vi "test4.vi"() -> ()   [LabVIEW 2020]
uses:
  <vilib>/Platform/TimedLoop/XDataNode/timing_clust.ctl
  <vilib>/Platform/TimedLoop/XDataNode/nitl_modes.ctl
  <vilib>/Platform/TimedLoop/XDataNode/wakeup.ctl
  37583fcc-cec8-480d-a6d0-1da09da3d0dd.vi
  <vilib>/platform/TimedLoop/XDataNode/XDataNode.xnode
  <vilib>/Platform/TimedLoop/XDataNode/XDNodeRunTimeDep.lvlib
panel:
  out "Tank":dbl(slide) scale=0.0..1.0
  out "Current XY":cluster{"X":dbl, "Y":dbl}
  out "XY Graph":cluster{dbl[], dbl[]}[](graph)
  out "Move Time":u32
  out "Distance":dbl
  out "Start Time":u32
  out "Start XY":cluster{"X":dbl, "Y":dbl}
  out "Target XY":cluster{"X":dbl, "Y":dbl}
  out "Stopped":bool
  in  "Stop":bool
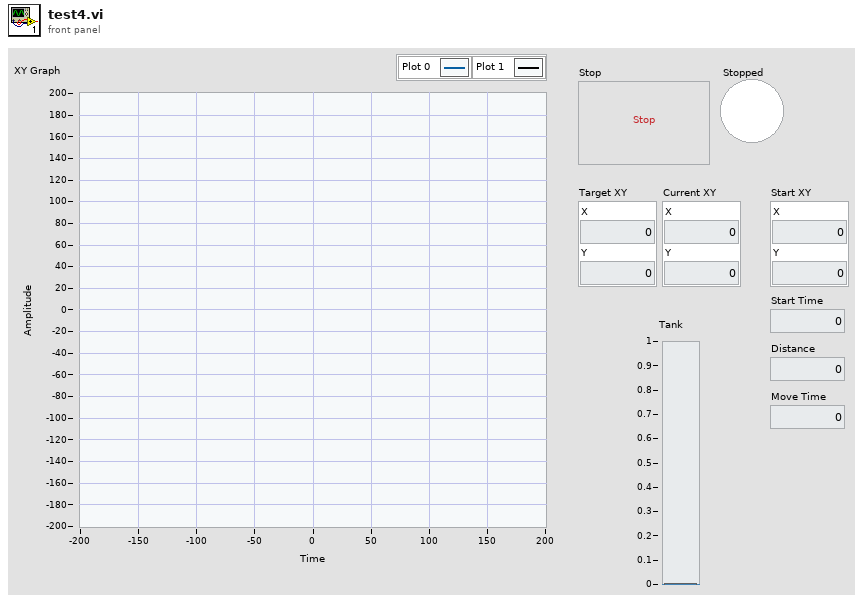
[diagram p1: front panel]
types:
  T1 = typedef "XDNodeRunTimeDep.lvlib/timing_clust.ctl" = cluster{"Expected End [f-1]":u64, "Actual End [f-1]":u64, "Finished Late? [f-1]":bool, "Expected End [i-1]":u64, "Actual End [i-1]":u64, "Finished Late? [i-1]":bool, "Expected Start [i]":u64, "Actual Start [i]":u64, "Expected Start [f]":u64, "Actual Start [f]":u64, "Source Name":string, "Structure Name":string, "Period":i64, "Deadline":i64, "Offset":i64, "Start":i64, "Priority":i32, "Timeout":i32, "Mode":T2, "Wakeup Reason":T3, "Error":errorcluster, "Source Type":string, "Secondary Source Type":string, "Global End Time":u64, "Global Start Time":u64, "Frame Duration":u64, "Iteration Duration":u64, "Assigned CPU":i32, "I/O Scan Engine Mode":u32}
  T2 = typedef "XDNodeRunTimeDep.lvlib/nitl_modes.ctl" = enum32{"No Change", "Process missed periods, maintain original phase", "Discard missed periods, maintain original phase", "Process missed periods, ignore original phase", "Discard missed periods, ignore original phase"}
  T3 = typedef "XDNodeRunTimeDep.lvlib/wakeup.ctl" = enum32{"Normal", "Aborted", "Asynchronous wakeup", "Timing source error", "Timed loop error", "Timeout"}
  T4 = typedef "LVPoint32TypeDef.ctl" = cluster{"Horizontal":i32, "Vertical":i32}
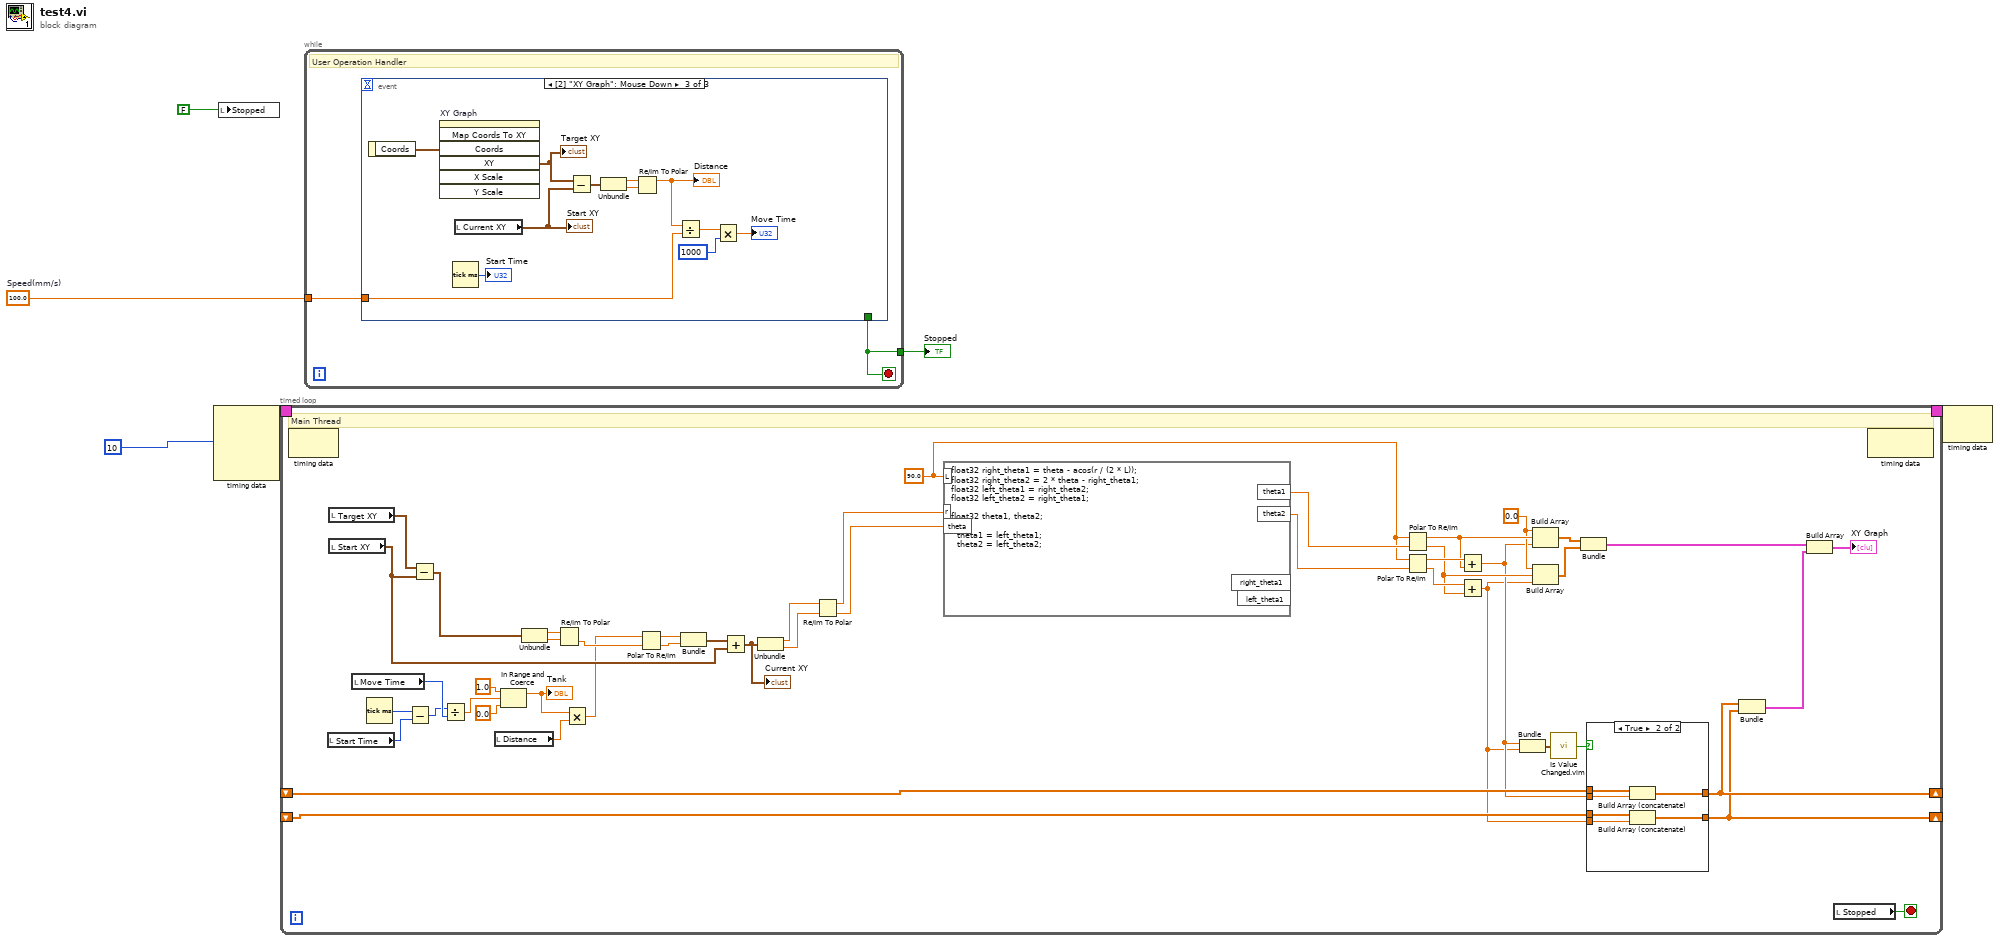
[diagram p0: block diagram]
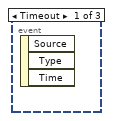
[diagram p3: hidden frame]
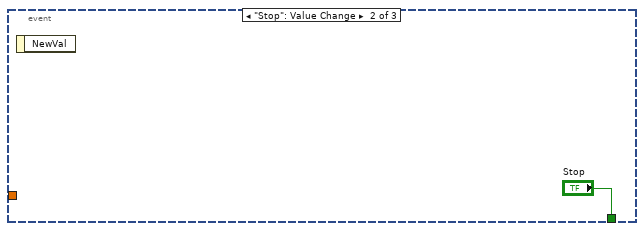
[diagram p4: hidden frame]
diagram:
  w1 = 100.0  # Speed(mm/s)
  n1 = node-c288(i64 10 ("Period")) -> (w6:T1)  [unwired: 3 in]
  n2 = local write "Stopped"(FALSE ("Stopped")) -> ()
  n3 = timed-loop {
    timing: w6 -> [_]
    timing-out: [_] -> w5
    shift-right: [w15] -> _
    shift-left: _ -> [w22]
    shift-right: [w14] -> _
    shift-left: _ -> [w21]
    stop <- w52 stop-if-true
    w27 = 0.0 ("element")
    w24 = 90.0 ("input variable")
    # "Main Thread"
    n4 = node-c288() -> ()  [unwired: 1 in, 1 out]
    n5 = local read "Start Time"() -> (w50:u32)
    n6 = local read "Target XY"() -> (w49:cluster{"X":dbl, "Y":dbl})
    n7 = local read "Start XY"() -> (w40:cluster{"X":dbl, "Y":dbl})
    n8 = local read "Move Time"() -> (w36:u32)
    n9 = Tick Count (ms)() -> (millisecond timer value=w51:u32)
    n10 = Subtract(x=w51, y=w50) -> (x-y=w11:u32)
    n11 = Subtract(x=w49, y=w40) -> (x-y=w47:cluster{"X":dbl, "Y":dbl})
    n12 = Divide(x=w11, y=w36) -> (x/y=w10:dbl)
    n13 = local read "Distance"() -> (w48:dbl)
    n14 = In Range and Coerce(upper limit=1.0 ("lower limit"), x=w10, lower limit=0.0) -> (coerced(x)=w7:dbl)  [unwired: 1 out]
    "Tank" <- w7
    n15 = Unbundle(w47) -> ("X"=w46:dbl, "Y"=w45:dbl)
    n16 = Re/Im To Polar(2:w45, 3:w46) -> (0:w44:dbl)  [unwired: 1 out]
    n17 = Multiply(x=w7, y=w48) -> (x*y=w35:dbl)
    n18 = Polar To Re/Im(2:w44, 3:w35) -> (0:w42:dbl, 1:w43:dbl)
    n19 = Bundle(w43, w42) -> (w41:cluster{dbl, dbl})  [unwired: 1 in]
    n20 = Add(x=w41, y=w40) -> (x+y=w23:cluster{dbl, dbl})
    "Current XY" <- w23
    n21 = Unbundle(w23) -> (w39:dbl, w38:dbl)
    n22 = Re/Im To Polar(2:w38, 3:w39) -> (0:w37:dbl, 1:w34:dbl)
    n23 = formula code="float32 right_theta1 = theta - acos(r / (2 * L));\nfloat32 right_theta2 = 2 * theta - right_theta1;\nfloat32 left_theta1 = right_theta2;\nfloat32 left_theta2 = right_theta1;\n\nfloat32 theta1, theta2;\n\n  theta1 = left_theta1;\n  theta2 = left_theta2;"("r"=w34, "theta"=w37, "L"=w24) -> ("theta1"=w26:sgl, "theta2"=w25:sgl)  [unwired: 2 out]
    n24 = Polar To Re/Im(2:w26, 3:w24) -> (0:w30:dbl, 1:w31:dbl)
    n25 = Polar To Re/Im(2:w25, 3:w24) -> (0:w32:dbl, 1:w33:dbl)
    n26 = Add(x=w33, y=w31) -> (x+y=w20:dbl)
    n27 = Add(x=w32, y=w30) -> (x+y=w19:dbl)
    n28 = Bundle(w20, w19) -> (w18:cluster{dbl, dbl})  [unwired: 1 in]
    n29 = Build Array(w27, w31, w20) -> (w29:dbl[])
    n30 = Build Array(w27, w30, w19) -> (w28:dbl[])
    n31 = call "Is Value Changed.vim"("value"=w18) -> ("changed or first call?"=w17:bool)
    n32 = Bundle(w29, w28) -> (w16:cluster{dbl[], dbl[]})  [unwired: 1 in]
    n33 = case shown="True" w17 {
      tunnel: w20 -> [_ w60]
      tunnel: w19 -> [_ w59]
      tunnel: [w54 w58] -> w15
      tunnel: [w53 w57] -> w14
      tunnel: w22 -> [w54 w56]
      tunnel: w21 -> [w53 w55]
      frame False {
      }
      frame True {
        n34 = Build Array (concatenate)(w56, w60) -> (w58:dbl[])
        n35 = Build Array (concatenate)(w55, w59) -> (w57:dbl[])
      }
    }
    n36 = Bundle(w15, w14) -> (w13:cluster{dbl[], dbl[]})  [unwired: 1 in]
    n37 = Build Array(w16, w13) -> (→"XY Graph":cluster{dbl[], dbl[]}[])
    n38 = local read "Stopped"() -> (w52:bool)
    n39 = node-c288() -> ()  [unwired: 1 in, 1 out]
  }
  n40 = while {
    tunnel: [w64] -> w4
    tunnel: w1 -> [w63]
    stop <- w64 stop-if-true
    # "User Operation Handler"
    n41 = event shown="[2] \"XY Graph\": Mouse Down" {
      selector: _ -> [_ _ _]
      dyn-events: _ -> [_ _ _]
      timeout: _ -> [_ _ _]
      tunnel: [_ "Stop" _] -> w64
      tunnel: w63 -> [_ _ w75]
      event Timeout {
        n42 = event-data() -> ()  [unwired: 1 in, 3 out]
      }
      event "Stop": Value Change {
        n43 = event-data() -> ()  [unwired: 1 in, 1 out]
      }
      event "XY Graph": Mouse Down {
        n44 = event-data() -> ("Coords"=w71:T4)  [unwired: 1 in]
        n45 = invoke on="XY Graph" class="XYGraph (strict)" method="Map Coords To XY"("Coords"=w71) -> ("XY"=w70:cluster{"X":dbl, "Y":dbl})  [unwired: 6 in, 6 out]
        "Target XY" <- w70
        n46 = Tick Count (ms)() -> (millisecond timer value=→"Start Time":u32)
        n47 = local read "Current XY"() -> (w69:cluster{"X":dbl, "Y":dbl})
        "Start XY" <- w69
        n48 = Subtract(x=w70, y=w69) -> (x-y=w68:cluster{"X":dbl, "Y":dbl})
        n49 = Unbundle(w68) -> ("X"=w67:dbl, "Y"=w66:dbl)
        n50 = Re/Im To Polar(2:w66, 3:w67) -> (1:w76:dbl)  [unwired: 1 out]
        "Distance" <- w76
        n51 = Divide(x=w76, y=w75) -> (x/y=w74:dbl)
        n52 = Multiply(x=w74, y=u32 1000 ("millisecond timer value")) -> (x*y=→"Move Time":dbl)
      }
    }
  }
  "Stopped" <- w4
  n53 = node-c288(w5) -> ()  [unwired: 1 out]
